vi "Limit Specification for UnEvenly Sampled Data (subVI).vi"(0 "Specification Cluster":cluster{"X":dbl[], "Y":dbl[]} {"Y" format="%#.6g"; "X" format="%#.6g"}, 1 "reset":bool, 7 "dx":dbl format="%#.6g", 9 "x0":dbl format="%#.6g", 11 "error in (no error)":errorcluster, 13 "X Values for Signal":dbl[](array[numeric]) format="%#.6g") -> (4 "Limit":cluster{"x0":dbl, "dx":dbl, "Y":dbl[]} {"Y" format="%#.6g"; "dx" format="%#.6g"; "x0" format="%#.6g"}, 15 "error out":errorcluster)   [LabVIEW 2023]
doc: "The Create Limit VI creates the limit as defined by the input array X and Y. The input array X contains the X axis values for the limit and the input array Y contains the Y axis values for the limits. The VI interpolates the data in the array Y at points x0, x0 + dx, x0 + 2dx and so on, where x0 = X[0]. The input Mask Type determines whether the mask that will be created is continuous or segmented.\n\nThe input x0 allows you to create a limit starting from an arbitrary point. If x0 is not connected, then the VI creates the limit starting from the first point in the X input array. If Reset is true, the VI creates a new limit. Else, it returns the limit created in the previous call."
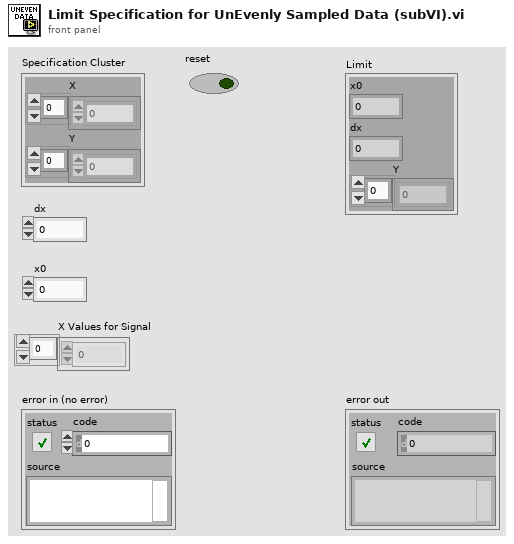
[diagram p1: front panel]
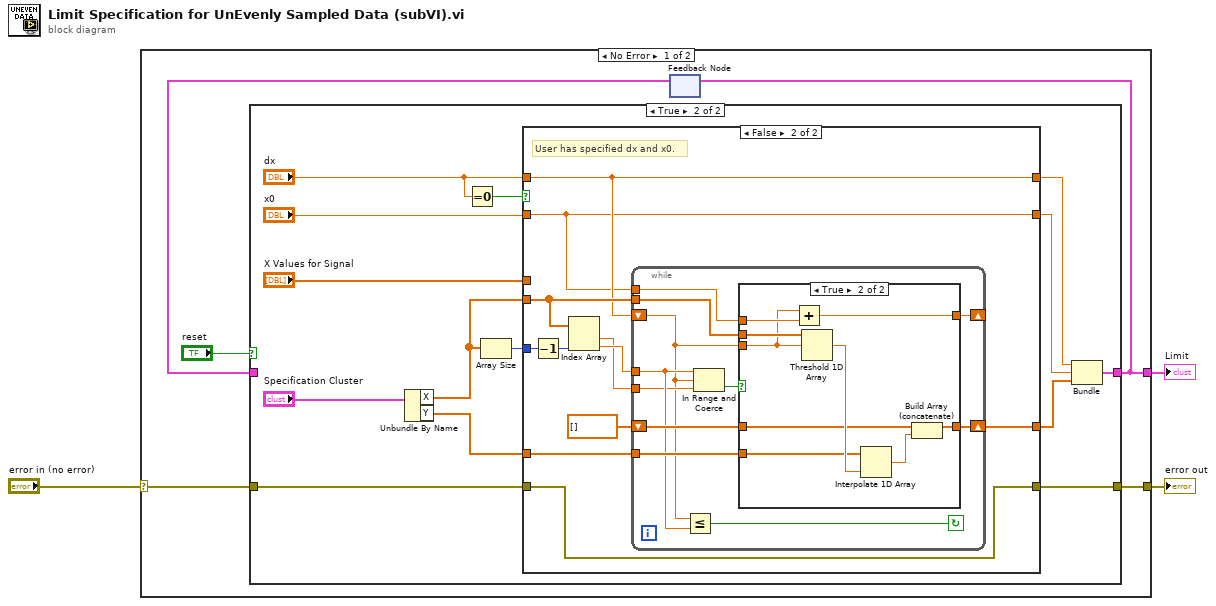
[diagram p0: block diagram]
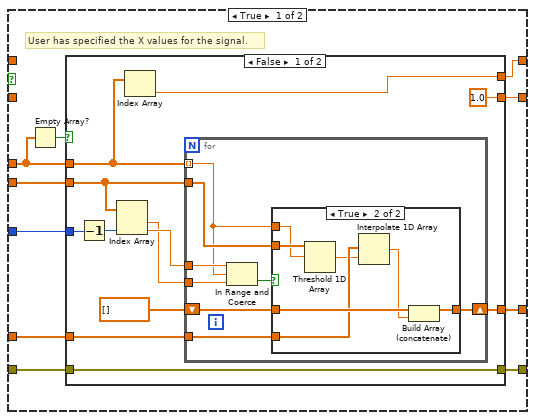
[diagram p3: hidden frame]
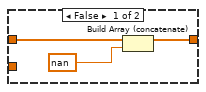
[diagram p4: hidden frame]
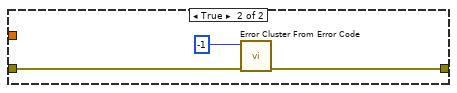
[diagram p5: hidden frame]
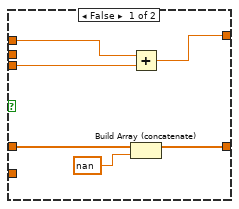
[diagram p6: hidden frame]
diagram:
  n1 = case shown="No Error" "error in (no error)" {
    selector: "error in (no error)" -> [w4 w105]
    tunnel: [w7 _] -> w1
    tunnel: [w8 w105] -> w2
    frame No Error {
      n2 = feedback #1() -> (w6:cluster{"dx":dbl, "x0":dbl, dbl[]})  [unwired: 1 in]
      n3 = case shown="True" "reset" {
        tunnel: [w10 w11] -> w7
        tunnel: w6 -> [w10 _]
        tunnel: w4 -> [w9 w16]
        tunnel: [w9 w15] -> w8
        frame False {
        }
        frame True {
          n4 = Unbundle By Name("Specification Cluster") -> ("X"=w20:dbl[], "Y"=w21:dbl[])
          n5 = Equal To 0?(x="dx") -> (x = 0?=w17:bool)
          n6 = Array Size(array=w20) -> (size(s)=w19:i32)
          n7 = case shown="False" w17 {
            tunnel: w21 -> [w34 w78]
            tunnel: w19 -> [w30 w77]
            tunnel: "x0" -> [_ w69]
            tunnel: [w33 w76] -> w12
            tunnel: "dx" -> [_ w74]
            tunnel: w20 -> [w31 w75]
            tunnel: "X Values for Signal" -> [w27 _]
            tunnel: [w32 w69] -> w13
            tunnel: [w25 w74] -> w14
            tunnel: w16 -> [w29 w70]
            tunnel: [w28 w70] -> w15
            frame True {
              # "User has specified the X values for the signal."
              n8 = Empty Array?(array=w27) -> (empty?=w26:bool)
              n9 = case shown="False" w26 {
                tunnel: w34 -> [w46 _]
                tunnel: [w44 _] -> w33
                tunnel: [1.0 _] -> w32
                tunnel: w27 -> [w43 _]
                tunnel: w31 -> [w42 _]
                tunnel: w30 -> [w41 _]
                tunnel: [w39 _] -> w25
                tunnel: w29 -> [w37 w67]
                tunnel: [w37 w66] -> w28
                frame False {
                  n10 = Decrement(x=w41) -> (x-1=w40:i32)
                  n11 = Index Array(array=w42, index #2=w40) -> (element #1=w36:dbl, element #2=w38:dbl)  [unwired: 1 in]
                  n12 = Index Array(array=w43) -> (element=w39:dbl)  [unwired: 1 in]
                  n13 = for {
                    shift-right: [w51] -> w44
                    shift-left: dbl[] [] -> [w54]
                    tunnel: w46 -> [w53]
                    tunnel: w42 -> [w52]
                    tunnel: w43 -> [w48] mode=indexing
                    tunnel: w38 -> [w49]
                    tunnel: w36 -> [w47]
                    n14 = In Range and Coerce(upper limit=w49, x=w48, lower limit=w47) -> (In Range?=w50:bool)  [unwired: 1 out]
                    n15 = case shown="True" w50 {
                      tunnel: [w57 w64] -> w51
                      tunnel: w54 -> [w56 w63]
                      tunnel: w53 -> [_ w62]
                      tunnel: w52 -> [_ w61]
                      tunnel: w48 -> [_ w59]
                      frame False {
                        n16 = Build Array (concatenate)(w56, nan ("Input Element")) -> (w57:dbl[])
                      }
                      frame True {
                        n17 = Threshold 1D Array(2:w59, 3:w61) -> (0:w58:dbl)  [unwired: 1 in]
                        n18 = Interpolate 1D Array(1:w58, 2:w62) -> (0:w60:dbl)
                        n19 = Build Array (concatenate)(w63, w60) -> (w64:dbl[])
                      }
                    }
                  }
                }
                frame True {
                  n20 = call <vilib>:"Error Cluster From Error Code.vi"("error in (no error)"=w67, "error code (0)"=-1 ("Error Code")) -> ("error out"=w66:errorcluster)  [unwired: 7 in]
                }
              }
            }
            frame False {
              # "User has specified dx and x0."
              n21 = Decrement(x=w77) -> (x-1=w73:i32)
              n22 = Index Array(array=w75, index #2=w73) -> (element #1=w68:dbl, element #2=w72:dbl)  [unwired: 1 in]
              n23 = while {
                tunnel: w68 -> [w81]
                tunnel: w75 -> [w84]
                tunnel: w78 -> [w85]
                tunnel: w69 -> [w88]
                tunnel: w72 -> [w82]
                shift-left: dbl[] [] -> [w86]
                shift-right: [w87] -> w76
                shift-left: w74 -> [w80]
                shift-right: [w89] -> _
                stop <- w83 continue-if-true
                n24 = Less Or Equal?(x=w80, y=w82) -> (x <= y?=w83:bool)
                n25 = In Range and Coerce(upper limit=w82, x=w80, lower limit=w81) -> (In Range?=w79:bool)  [unwired: 1 out]
                n26 = case shown="True" w79 {
                  tunnel: [w93 w103] -> w87
                  tunnel: w86 -> [w95 w100]
                  tunnel: w80 -> [w91 w96]
                  tunnel: [w92 w101] -> w89
                  tunnel: w88 -> [w90 w102]
                  tunnel: w85 -> [_ w98]
                  tunnel: w84 -> [_ w97]
                  frame False {
                    n27 = Add(x=w90, y=w91) -> (x+y=w92:dbl)
                    n28 = Build Array (concatenate)(w95, nan ("Input Element")) -> (w93:dbl[])
                  }
                  frame True {
                    n29 = Add(x=w96, y=w102) -> (x+y=w101:dbl)
                    n30 = Threshold 1D Array(2:w96, 3:w97) -> (0:w104:dbl)  [unwired: 1 in]
                    n31 = Interpolate 1D Array(1:w104, 2:w98) -> (0:w99:dbl)
                    n32 = Build Array (concatenate)(w100, w99) -> (w103:dbl[])
                  }
                }
              }
            }
          }
          n33 = Bundle("dx"=w14, "x0"=w13, w12) -> (w11:cluster{"dx":dbl, "x0":dbl, dbl[]})  [unwired: 1 in]
        }
      }
      n34 = feedback-in #1(w7) -> ()
    }
    frame Error {
    }
  }
  "error out" <- w2
  "Limit" <- w1
